vi "strip_path.vi"(11 "path":string) -> (2 "name":string, 3 "stripped_path":string)   [LabVIEW 2015, in "lv-dropbox.lvlib"]
uses:
  lv-dropbox.lvlib
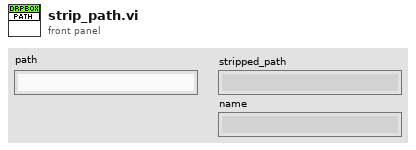
[diagram p1: front panel]
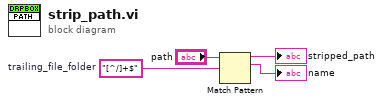
[diagram p0: block diagram]
diagram:
  w3 = "[^/]+$"  # trailing_file_folder
  n1 = Match Pattern(string="path", regular expression=w3) -> (before substring=→"stripped_path":string, match substring=→"name":string)  [unwired: 1 in, 2 out]
